vi "RT Driver VI.vi"(6 "Device Clock":string, 9 "Device Inputs FIFO":refnum<k33>, 10 "Device Outputs FIFO":refnum<k33>, 11 "Device Reference":T1 format="%.0x") -> ()   [LabVIEW 2013, in "PWM Engine.lvlib"]
uses:
  PWM Engine.lvlib
  <vilib>/NI Veristand/Custom Device API/Custom Device Item Ref.ctl
  <vilib>/NI Veristand/Custom Device API/Custom Device Channel Type.ctl
  <vilib>/Platform/TimedLoop/XDataNode/timing_clust.ctl
  <vilib>/Platform/TimedLoop/XDataNode/nitl_modes.ctl
  <vilib>/Platform/TimedLoop/XDataNode/wakeup.ctl
  <vilib>/FPGAPlugInAG/Dynamic/niLvFpga_Close_Dynamic.vi
  <vilib>/Utility/error.llb/Simple Error Handler.vi
  <vilib>/NI Veristand/Custom Device Tools/Custom Device Utility Library/NI VeriStand - Print Debug String.vi
  <vilib>/Platform/TimedLoop/XDataNode/XDataNode.xnode
  <vilib>/rvi/interface/nirviCloseFPGA/nirviCloseFPGA.xnode
  <vilib>/NI Veristand/Custom Device API/Custom Device API.lvlib
  <vilib>/NI Veristand/Custom Device Tools/Custom Device Utility Library/Custom Device Utility Library.lvlib
  <vilib>/Platform/TimedLoop/XDataNode/XDNodeRunTimeDep.lvlib
panel:
  in  "Initialization Status Notifier":refnum<notifier>
  in  "Status Notifier":refnum<notifier>
  # "Custom Device Template\nv1.0"
  # "Use this template as a starting point for creating a custom device code module. The input controls shown here are specially named controls that the system will use to provide the device loop with data. The controls are not required for the device loop to run. For instance, if the device doesn't produce any output data, then you don't need the Device Outputs FIFO control. If you do use these controls, however, they need to have these exact names to be functional."
  # "The optional status notifier element is used to notify the RT engine of the last state of the custom device, and to indicate the device has completed execution. If this control is not used, a default No Error value is returned to the system when the device finishes execution.\n\nNote: This error state is not checked until the system shuts down. Use an output status channel to send more immediate status values to the system."
  # "This optional input can be used to send the VeriStand Engine the final status of the custom device initalization process. If this control exists on the custom device front panel, the VeriStand Engine will wait for a status update before starting up. If the custom device reports an error, that will abort the execution of the current configuration in the VeriStand Engine.\n\nThis control can be deleted if the custom device does not need to send the initialization status update."
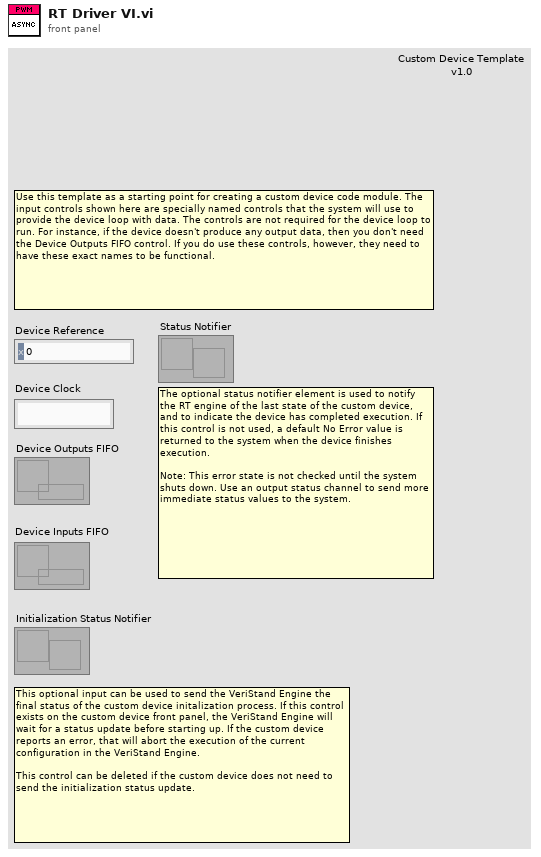
[diagram p1: front panel]
types:
  T1 = typedef "Custom Device API.lvlib/Custom Device Item Ref.ctl" = u64
  T2 = typedef "Custom Device API.lvlib/Custom Device Channel Type.ctl" = enum16{"Input", "Output"}
  T3 = typedef "PWM Shared.lvlib/PWM data(RT).ctl" = cluster{"PWM out(added)":T4[], "PWM out(not added)":T4[], "PWM in(added)":T5[]}
  T4 = typedef "PWM Shared.lvlib/PWM out info(RT).ctl" = cluster{"buffer index (Duty cycle)":i32, "buffer index (Frequency)":i32, "Init Frequency":dbl, "Init Duty Cycle":dbl, "PWM out ctl ref":refnum<k20>}
  T5 = typedef "PWM Shared.lvlib/PWM in info(RT).ctl" = cluster{"buffer index (Duty cycle)":i32, "buffer index (Frequency)":i32, "PWM in ctl ref":refnum<k20>}
  T6 = typedef "XDNodeRunTimeDep.lvlib/timing_clust.ctl" = cluster{"Expected End [f-1]":u64, "Actual End [f-1]":u64, "Finished Late? [f-1]":bool, "Expected End [i-1]":u64, "Actual End [i-1]":u64, "Finished Late? [i-1]":bool, "Expected Start [i]":u64, "Actual Start [i]":u64, "Expected Start [f]":u64, "Actual Start [f]":u64, "Source Name":string, "Structure Name":string, "Period":i64, "Deadline":i64, "Offset":i64, "Start":i64, "Priority":i32, "Timeout":i32, "Mode":T7, "Wakeup Reason":T8, "Error":errorcluster, "Source Type":string, "Secondary Source Type":string, "Global End Time":u64, "Global Start Time":u64, "Frame Duration":u64, "Iteration Duration":u64, "Assigned CPU":i32, "I/O Scan Engine Mode":u32}
  T7 = typedef "XDNodeRunTimeDep.lvlib/nitl_modes.ctl" = enum32{"No Change", "Process missed periods, maintain original phase", "Discard missed periods, maintain original phase", "Process missed periods, ignore original phase", "Discard missed periods, ignore original phase"}
  T8 = typedef "XDNodeRunTimeDep.lvlib/wakeup.ctl" = enum32{"Normal", "Aborted", "Asynchronous wakeup", "Timing source error", "Timed loop error", "Timeout"}
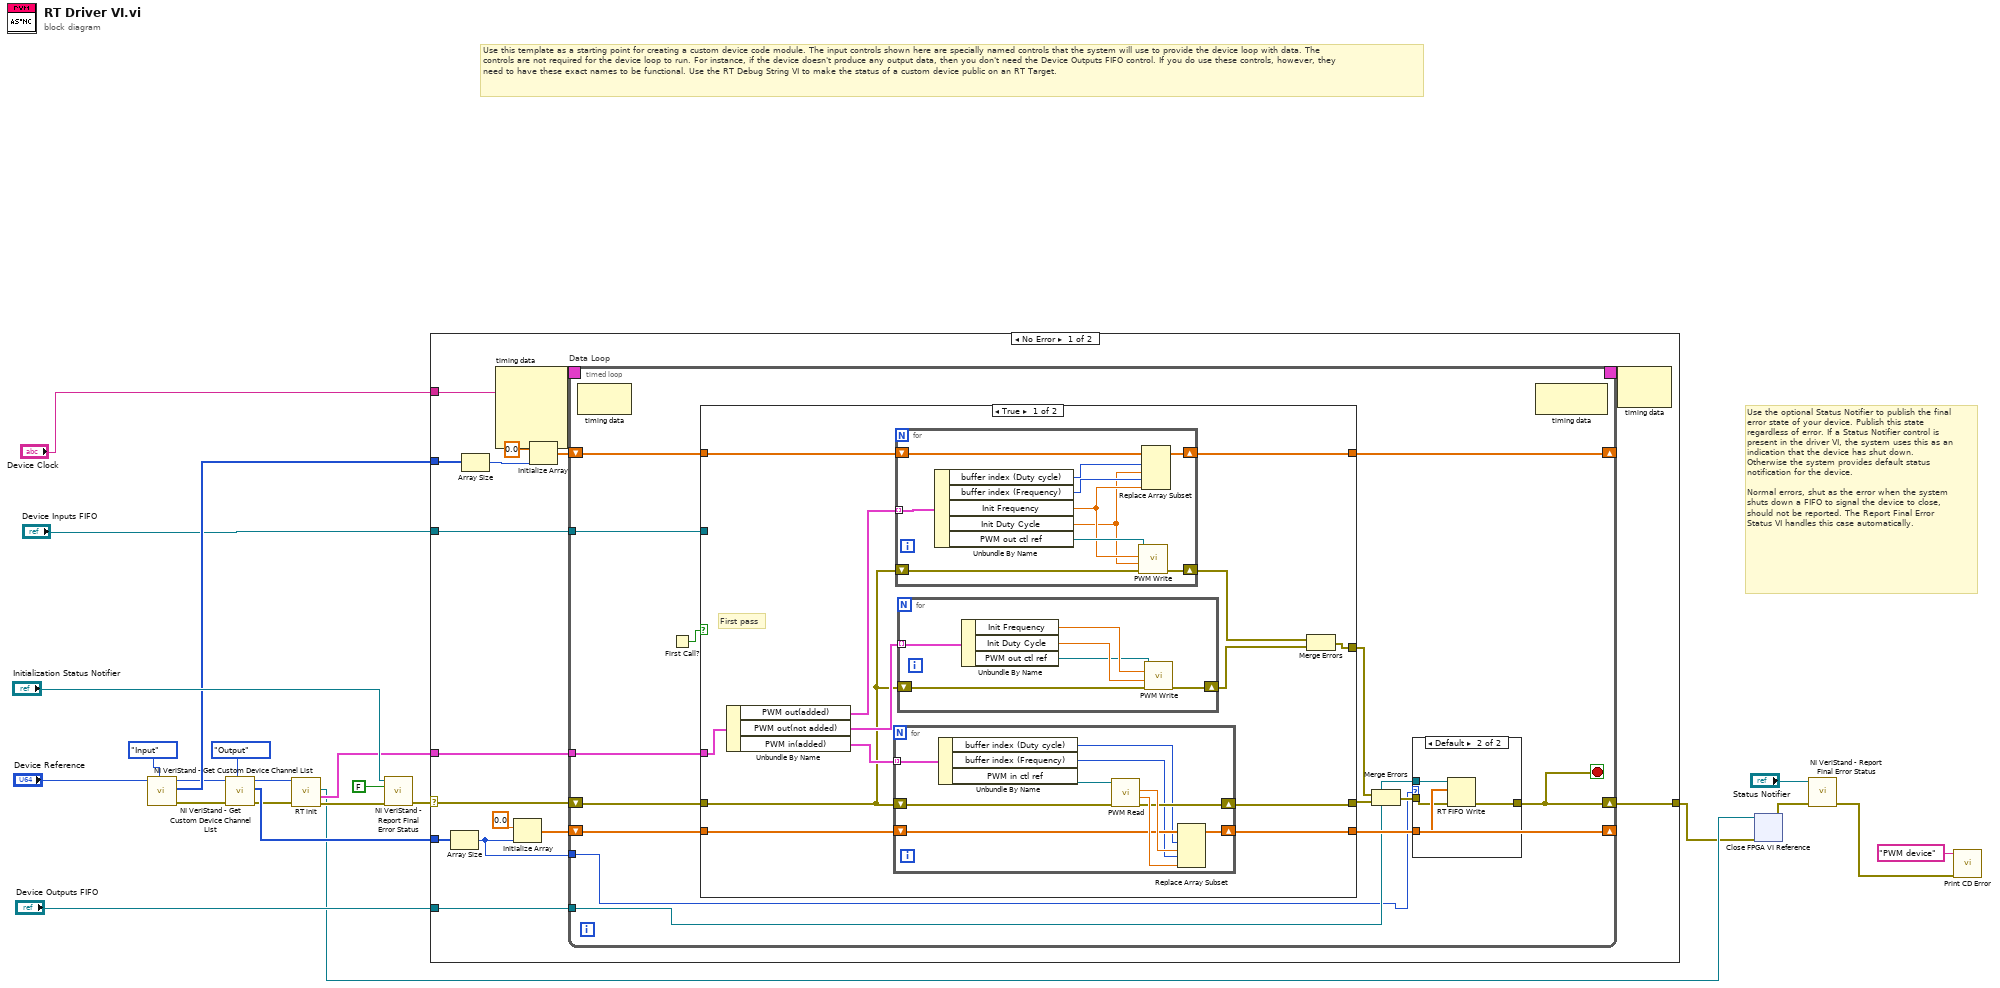
[diagram p0: block diagram]
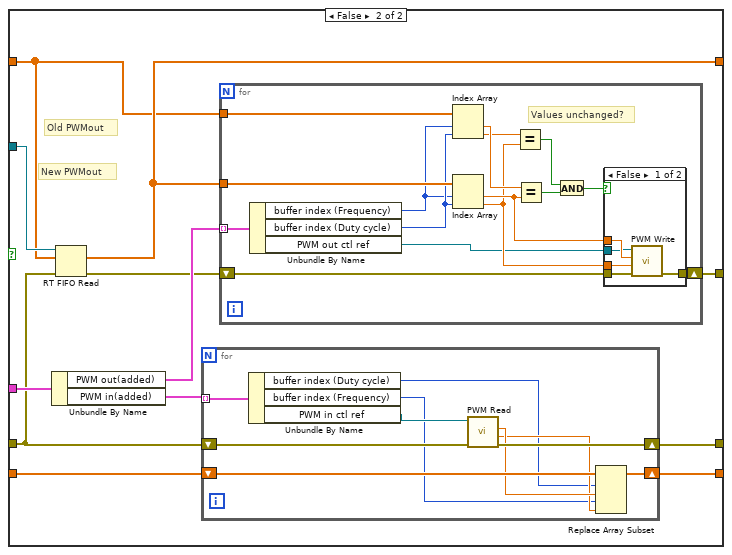
[diagram p3: hidden frame]
diagram:
  # "Use the optional Status Notifier to publish the final error state of your device. Publish this state regardless of error. If a Status Notifier control is present in the driver VI, the system uses this as an indication that the device has shut down. Otherwise the system provides default status notification for the device.\n\nNormal errors, shut as the error when the system shuts down a FIFO to signal the device to close, should not be reported. The Report Final Error Status VI handles this case automatically."
  # "Use this template as a starting point for creating a custom device code module. The input controls shown here are specially named controls that the system will use to provide the device loop with data. The controls are not required for the device loop to run. For instance, if the device doesn't produce any output data, then you don't need the Device Outputs FIFO control. If you do use these controls, however, they need to have these exact names to be functional. Use the RT Debug String VI to make the status of a custom device public on an RT Target."
  n1 = call <vilib>:"NI VeriStand - Get Custom Device Channel List.vi"("Channel Type"=Custom_Device_Channel_Type."Input", "Device Ref in"="Device Reference") -> ("error out"=w14:errorcluster, "Specified Channel Ref List"=w21:T1[], "Device Ref out"=w15:T1)  [unwired: 1 in, 6 out]
  n2 = call <vilib>:"NI VeriStand - Get Custom Device Channel List.vi"("Channel Type"=Custom_Device_Channel_Type."Output", "error in (no error)"=w14, "Device Ref in"=w15) -> ("error out"=w11:errorcluster, "Specified Channel Ref List"=w22:T1[], "Device Ref out"=w9:T1)  [unwired: 6 out]
  n3 = call "RT init.vi"("error in (no error)"=w11, "Device Reference"=w9) -> ("error out"=w10:errorcluster, "PWM data"=w17:T3, "Bitfile Ref"=w4:refnum<k20>)  [unwired: 6 in, 1 out]
  n4 = call <vilib>:"NI VeriStand - Report Final Error Status.vi"("error in (no error)"=w10, "Filter FIFO & Shutdown Errors (T)"=FALSE ("Filter FIFO Errors (T)"), "Status Notifier"="Initialization Status Notifier") -> ("error out"=w19:errorcluster)  [unwired: 8 out]
  n5 = case shown="No Error" w19 {
    selector: w19 -> [w30 w147]
    tunnel: "Device Inputs FIFO" -> [w39 _]
    tunnel: "Device Outputs FIFO" -> [w38 _]
    tunnel: w22 -> [w33 _]
    tunnel: w21 -> [w32 _]
    tunnel: [w29 w147] -> w3
    tunnel: w17 -> [w31 _]
    tunnel: "Device Clock" -> [w25 _]
    frame No Error {
      n6 = Array Size(array=w33) -> (size(s)=w24:i32)
      n7 = Array Size(array=w32) -> (size(s)=w28:i32)
      n8 = node-c288(w25) -> (w27:T6)  [unwired: 3 in]
      n9 = Initialize Array(0.0 ("element"), w24) -> (w34:dbl[])
      n10 = Initialize Array(0.0 ("element"), w28) -> (w35:dbl[])
      n11 = timed-loop "Data Loop" {
        shift-right: [w53] -> _
        shift-left: w34 -> [w46]
        shift-right: [w41] -> w29
        shift-left: w30 -> [w47]
        shift-right: [w51] -> _
        shift-left: w35 -> [w52]
        tunnel: w39 -> [w50]
        tunnel: w38 -> [w49]
        tunnel: w31 -> [w48]
        timing: w27 -> [_]
        timing-out: [_] -> w26
        tunnel: w24 -> [w40]
        stop <- w41 stop-if-true
        n12 = node-c288() -> ()  [unwired: 1 in, 1 out]
        n13 = First Call?() -> (First Call?: T/F=w44:bool)
        n14 = case shown="True" w44 {
          tunnel: w48 -> [w71 w109]
          tunnel: w46 -> [w69 w107]
          tunnel: w47 -> [w64 w98]
          tunnel: [w63 w99] -> w53
          tunnel: w52 -> [w66 w100]
          tunnel: [w65 w101] -> w51
          tunnel: [w62 w105] -> w42
          tunnel: [w59 w104] -> w45
          tunnel: w50 -> [_ w102]
          frame True {
            # "First pass"
            n15 = Unbundle By Name(w71) -> ("PWM out(added)"=w67:T4[], "PWM out(not added)"=w68:T4[], "PWM in(added)"=w70:T5[])
            n16 = for {
              tunnel: w70 -> [w97] mode=indexing
              shift-right: [w96] -> w63
              shift-left: w69 -> [w93]
              shift-right: [w91] -> w62
              shift-left: w64 -> [w92]
              n17 = Unbundle By Name(w97) -> ("buffer index (Duty cycle)"=w89:i32, "buffer index (Frequency)"=w88:i32, "PWM in ctl ref"=w90:refnum<k20>)
              n18 = call "PWM Read.vi"("error in"=w92, "FPGA Interface"=w90) -> ("error out"=w91:errorcluster, "Frequency"=w94:dbl, "Duty Cycle"=w95:dbl)  [unwired: 7 in]
              n19 = Replace Array Subset(array=w93, new element #1=w95, index #1=w89, new element #2=w94, index #2=w88) -> (w96:dbl[])
            }
            n20 = for {
              shift-right: [w80] -> w61
              shift-left: w64 -> [w81]
              tunnel: w67 -> [w79] mode=indexing
              shift-right: [w78] -> w65
              shift-left: w66 -> [w77]
              n21 = Unbundle By Name(w79) -> ("buffer index (Duty cycle)"=w75:i32, "buffer index (Frequency)"=w74:i32, "Init Frequency"=w73:dbl, "Init Duty Cycle"=w72:dbl, "PWM out ctl ref"=w76:refnum<k20>)
              n22 = call "PWM Write.vi"("error in"=w81, "Duty Cycle"=w72, "Frequency"=w73, "FPGA Interface"=w76) -> ("error out"=w80:errorcluster)  [unwired: 7 in]
              n23 = Replace Array Subset(array=w77, new element #1=w72, index #1=w75, new element #2=w73, index #2=w74) -> (w78:dbl[])
            }
            n24 = for {
              tunnel: w68 -> [w87] mode=indexing
              shift-right: [w85] -> w60
              shift-left: w64 -> [w86]
              n25 = Unbundle By Name(w87) -> ("Init Frequency"=w83:dbl, "Init Duty Cycle"=w84:dbl, "PWM out ctl ref"=w82:refnum<k20>)
              n26 = call "PWM Write.vi"("error in"=w86, "Duty Cycle"=w84, "Frequency"=w83, "FPGA Interface"=w82) -> ("error out"=w85:errorcluster)  [unwired: 7 in]
            }
            n27 = Merge Errors(w61, w60) -> (w59:errorcluster)
          }
          frame False {
            # "New PWMout"
            # "Old PWMout"
            n28 = Unbundle By Name(w109) -> ("PWM out(added)"=w106:T4[], "PWM in(added)"=w108:T5[])
            n29 = RT FIFO Read(0:w102, 1:w100, 3:w98) -> (9:w101:dbl[], 11:w103:errorcluster)  [unwired: 1 in, 3 out]
            n30 = for {
              tunnel: w108 -> [w138] mode=indexing
              shift-right: [w140] -> w99
              shift-left: w107 -> [w136]
              shift-right: [w139] -> w105
              shift-left: w98 -> [w135]
              n31 = Unbundle By Name(w138) -> ("buffer index (Duty cycle)"=w132:i32, "buffer index (Frequency)"=w131:i32, "PWM in ctl ref"=w137:refnum<k20>)
              n32 = call "PWM Read.vi"("error in"=w135, "FPGA Interface"=w137) -> ("error out"=w139:errorcluster, "Frequency"=w133:dbl, "Duty Cycle"=w134:dbl)  [unwired: 7 in]
              n33 = Replace Array Subset(array=w136, new element #1=w134, index #1=w132, new element #2=w133, index #2=w131) -> (w140:dbl[])
            }
            n34 = for {
              shift-right: [w123] -> w104
              shift-left: w103 -> [w124]
              tunnel: w106 -> [w122] mode=indexing
              tunnel: w101 -> [w120]
              tunnel: w100 -> [w121]
              # "Values unchanged?"
              n35 = Unbundle By Name(w122) -> ("buffer index (Frequency)"=w110:i32, "buffer index (Duty cycle)"=w111:i32, "PWM out ctl ref"=w112:refnum<k20>)
              n36 = Index Array(array=w121, index #1=w110, index #2=w111) -> (element #1=w119:dbl, element #2=w118:dbl)
              n37 = Index Array(array=w120, index #1=w110, index #2=w111) -> (element #1=w114:dbl, element #2=w113:dbl)
              n38 = Equal?(x=w118, y=w113) -> (x = y?=w117:bool)
              n39 = Equal?(x=w119, y=w114) -> (x = y?=w116:bool)
              n40 = And(x=w117, y=w116) -> (x .and. y?=w115:bool)
              n41 = case shown="False" w115 {
                tunnel: w124 -> [w129 w130]
                tunnel: [w128 w130] -> w123
                tunnel: w114 -> [w127 _]
                tunnel: w113 -> [w126 _]
                tunnel: w112 -> [w125 _]
                frame False {
                  n42 = call "PWM Write.vi"("error in"=w129, "Duty Cycle"=w126, "Frequency"=w127, "FPGA Interface"=w125) -> ("error out"=w128:errorcluster)  [unwired: 7 in]
                }
                frame True {
                }
              }
            }
          }
        }
        n43 = Merge Errors(w45, w42) -> (w43:errorcluster)
        n44 = case shown="Default" w40 {
          tunnel: w53 -> [_ w58]
          tunnel: w49 -> [_ w57]
          tunnel: w43 -> [w54 w56]
          tunnel: [w54 w55] -> w41
          frame 0 {
          }
          frame Default {
            n45 = RT FIFO Write(0:w57, 1:w58, 3:w56) -> (11:w55:errorcluster)  [unwired: 2 in, 3 out]
          }
        }
        n46 = node-c288() -> ()  [unwired: 1 in, 1 out]
      }
      n47 = node-c288(w26) -> ()  [unwired: 1 out]
    }
    frame Error {
    }
  }
  n48 = xnode "Close FPGA VI Reference"("FPGA VI Reference In"=w4, "error in"=w3) -> ("error out"=w5:errorcluster)
  n49 = call <vilib>:"NI VeriStand - Report Final Error Status.vi"("error in (no error)"=w5, "Status Notifier"="Status Notifier") -> ("error out"=w1:errorcluster)  [unwired: 1 in, 8 out]
  n50 = call "Print CD Error.vi"("error in"=w1, "Your code's public name"="PWM device") -> ()  [unwired: 8 in, 1 out]
